vi "xijk_calc_other_parameters.vi"(7 "Settings":T1={"search parameters"={"Paths"={"Path: Excitation filters"=path "", "Path: Dicroic filters"=path "", "Path: Emission filters"=path "", "Path reget"=path ""}, "table excitation"=[], "table dicroics"=[], "table emission"=[], "Integers"={"Select result number"=1}, "boolean selector array"=[], "table for calculation automagic"=[]}, "output cluster"={"Booleans"={"Unknown detector"=FALSE, "Dual band filters"=FALSE, "Dual emission by cubes"=FALSE, "FRET"=FALSE}, "Integers"={"Light source"=0, "Number of fluorophores"=0, "Wavelength of laser (nm) 1"=0, "Broadness of laser (nm) 1"=0.0, "Wavelength of laser (nm) 2"=0, "Broadness of laser (nm) 2"=0.0, "Template"=1}, "Doubles"={"Molar extinction 1"=1.0, "Molar extinction 2"=1.0, "Quantum efficiency 1"=1.0, "Quantum efficiency 2"=1.0}}, "output cluster 2"={"Excitation filter 1"=path "", "Dichroic filter 1"=path "", "Emission filter 1"=path "", "Excitation filter 2"=path "", "Dichroic filter 2"=path "", "Emission filter 2"=path "", "Extra em filter 1"=path "", "Extra em filter 2"=path "", "Light source file"=path "", "Fluorophore absorption 1"=path "", "Fluorophore emission 1"=path "", "Fluorophore absorption 2"=path "", "Fluorophore emission 2"=path "", "Detector"=path ""}, "cluster de sortie"={"Excitation filter_x"=[], "Excitation filter_y"=[], "Dichroic filter_x"=[], "Dichroic filter_y"=[], "Emission filter_x"=[], "Emission filter_y"=[], "Excitation filter_x 2"=[], "Excitation filter_y 2"=[], "Dichroic filter_x 2"=[], "Dichroic filter_y 2"=[], "Emission filter_x 2"=[], "Emission filter_y 2"=[], "Extra em filter_x 1"=[], "Extra em filter_y 1"=[], "Extra em filter_x 1"=[], "Extra em filter_y 2"=[], "Light source_x"=[], "Light source_y"=[], "Detector_x"=[], "Detector_y"=[], "Fluorophore absorption_x"=[], "Fluorophore absorption_y"=[], "Fluorophore emission_x"=[], "Fluorophore emission_y"=[], "Fluorophore absorption_x 2"=[], "Fluorophore absorption_y 2"=[], "Fluorophore emission_x 2"=[], "Fluorophore emission_y 2"=[], "laser_x"=[], "laser_y"=[], "laser_x 2"=[], "laser_y 2"=[], "quantum efficiency factor 1"=0.0, "quantum efficiency factor 2"=0.0, "lamp scaling factor"=0.0}, "Xijk output cluster"={"Xijk 111"=0.0, "Xijk 112"=0.0, "Xijk 121"=0.0, "Xijk 122"=0.0, "Xijk 211"=0.0, "Xijk 212"=0.0, "Xijk 221"=0.0, "Xijk 222"=0.0, "Eijk 111"=0.0, "Eijk 112"=0.0, "Eijk 121"=0.0, "Eijk 122"=0.0, "Eijk 211"=0.0, "Eijk 212"=0.0, "Eijk 221"=0.0, "Eijk 222"=0.0}, "GUI configuration"={"axes in"={"min x-axis excitation"=300, "max x-axis excitation"=800, "min x-axis emission"=300, "max x-axis emission"=800, "precision of results"=2}, "plot colors in"={"Lanscape Portrait"=FALSE, "Plot logarithmic"=FALSE, "Ex/Em filters double"=FALSE, "Line colors"=[16734569, 56375, 16711916, 5896447, 16448250, 56375]}}, "references"={"Excitation filter 1 ref"=refnum, "Dichroic filter 1 ref"=refnum, "Emission filter 1 ref"=refnum, "Excitation filter 2 ref"=refnum, "Dichroic filter 2 ref"=refnum, "Emission filter 2 ref"=refnum, "Extra em filter 1 ref"=refnum, "Extra em filter 2 ref"=refnum, "Light source file ref"=refnum, "Fluorophore absorption 1 ref"=refnum, "Fluorophore emission 1 ref"=refnum, "Fluorophore absorption 2 ref"=refnum, "Fluorophore emission 2 ref"=refnum, "Detector ref"=refnum}} {"GUI configuration"."axes in"."precision of results" max=8 step=1}, 8 "Effective spectral emission 2":sgl[](array[numeric]), 9 "Effective spectral excitation 2":sgl[](array[numeric]), 10 "Effective spectral emission 1":sgl[](array[numeric]), 11 "Effective spectral excitation 1":sgl[](array[numeric])) -> (3 "array out":dbl[](array[numeric]))   [LabVIEW 2009]
uses:
  Type Def/settings.ctl
  Type Def/search_parameters.ctl
  Type Def/spectra_parameters.ctl
  Type Def/filepath.ctl
  Type Def/spectrum_table_control.ctl
  Type Def/xijk_cluster.ctl
  Type Def/configuration_cluster.ctl
  Type Def/axis_parameters.ctl
  Type Def/color_parameters.ctl
  Type Def/control_references_cluster.ctl
  <vilib>/Analysis/8numeric.llb/1D Numeric Integration.vi
  <vilib>/Analysis/NI_AALPro.lvlib
panel:
  out "% red emission in green channel":dbl
  out "spectral overlap efficiency":dbl
  out "% green emission in red channel":dbl
  out "excite %\nabsorption 2":dbl
  out "capture %\nemission 2":dbl
  out "excitation light bleed through 2":dbl caption="excitation light bleed through" format="%0.3e"
  out "excite %\nabsorption":dbl
  out "capture %\nemission":dbl
  out "excitation light bleed through":dbl format="%0.3e"
  # "Dichroic"
  # "Ex/Em filter"
  # "Fluorophore 1"
  # "Fluorophore 2"
  # "Laser /\nextra Em filter"
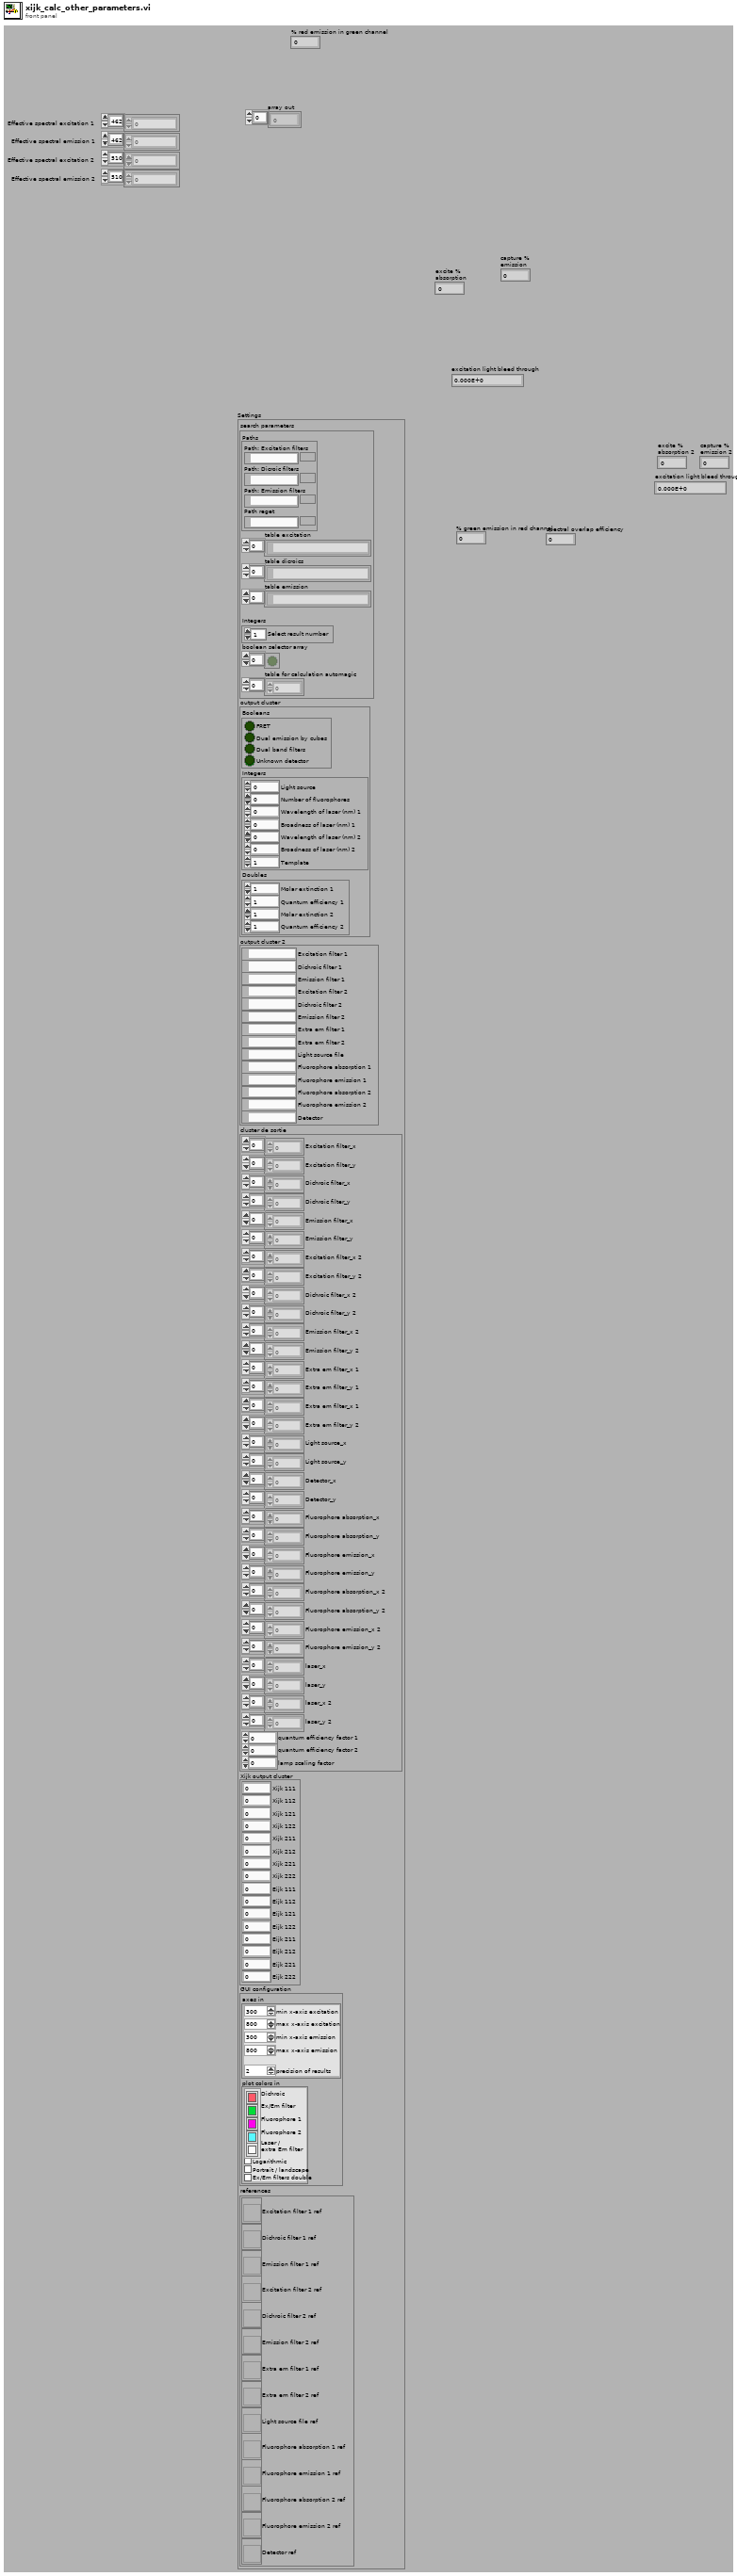
[diagram p1: front panel]
types:
  T1 = typedef "settings.ctl" = cluster{"search parameters":T2, "output cluster":T3, "output cluster 2":T4, "cluster de sortie":T5, "Xijk output cluster":T6, "GUI configuration":T7, "references":T10}
  T2 = typedef "search_parameters.ctl" = cluster{"Paths":cluster{"Path: Excitation filters":path, "Path: Dicroic filters":path, "Path: Emission filters":path, "Path reget":path}, "table excitation":path[], "table dicroics":path[], "table emission":path[], "Integers":cluster{"Select result number":u32}, "boolean selector array":bool[], "table for calculation automagic":i32[]}
  T3 = typedef "spectra_parameters.ctl" = cluster{"Booleans":cluster{"Unknown detector":bool, "Dual band filters":bool, "Dual emission by cubes":bool, "FRET":bool}, "Integers":cluster{"Light source":u16, "Number of fluorophores":u16, "Wavelength of laser (nm) 1":u16, "Broadness of laser (nm) 1":sgl, "Wavelength of laser (nm) 2":u16, "Broadness of laser (nm) 2":sgl, "Template":u16}, "Doubles":cluster{"Molar extinction 1":sgl, "Molar extinction 2":sgl, "Quantum efficiency 1":sgl, "Quantum efficiency 2":sgl}}
  T4 = typedef "filepath.ctl" = cluster{"Excitation filter 1":path, "Dichroic filter 1":path, "Emission filter 1":path, "Excitation filter 2":path, "Dichroic filter 2":path, "Emission filter 2":path, "Extra em filter 1":path, "Extra em filter 2":path, "Light source file":path, "Fluorophore absorption 1":path, "Fluorophore emission 1":path, "Fluorophore absorption 2":path, "Fluorophore emission 2":path, "Detector":path}
  T5 = typedef "spectrum_table_control.ctl" = cluster{"Excitation filter_x":i16[], "Excitation filter_y":sgl[], "Dichroic filter_x":i16[], "Dichroic filter_y":sgl[], "Emission filter_x":i16[], "Emission filter_y":sgl[], "Excitation filter_x 2":i16[], "Excitation filter_y 2":sgl[], "Dichroic filter_x 2":i16[], "Dichroic filter_y 2":sgl[], "Emission filter_x 2":i16[], "Emission filter_y 2":sgl[], "Extra em filter_x 1":i16[], "Extra em filter_y 1":sgl[], "Extra em filter_x 1":i16[], "Extra em filter_y 2":sgl[], "Light source_x":i16[], "Light source_y":sgl[], "Detector_x":i16[], "Detector_y":sgl[], "Fluorophore absorption_x":i16[], "Fluorophore absorption_y":sgl[], "Fluorophore emission_x":i16[], "Fluorophore emission_y":sgl[], "Fluorophore absorption_x 2":i16[], "Fluorophore absorption_y 2":sgl[], "Fluorophore emission_x 2":i16[], "Fluorophore emission_y 2":sgl[], "laser_x":i16[], "laser_y":sgl[], "laser_x 2":i16[], "laser_y 2":sgl[], "quantum efficiency factor 1":sgl, "quantum efficiency factor 2":sgl, "lamp scaling factor":sgl}
  T6 = typedef "xijk_cluster.ctl" = cluster{"Xijk 111":sgl, "Xijk 112":sgl, "Xijk 121":sgl, "Xijk 122":sgl, "Xijk 211":sgl, "Xijk 212":sgl, "Xijk 221":sgl, "Xijk 222":sgl, "Eijk 111":sgl, "Eijk 112":sgl, "Eijk 121":sgl, "Eijk 122":sgl, "Eijk 211":sgl, "Eijk 212":sgl, "Eijk 221":sgl, "Eijk 222":sgl}
  T7 = typedef "configuration_cluster.ctl" = cluster{"axes in":T8, "plot colors in":T9}
  T8 = typedef "axis_parameters.ctl" = cluster{"min x-axis excitation":u16, "max x-axis excitation":u16, "min x-axis emission":u16, "max x-axis emission":u16, "precision of results":u8}
  T9 = typedef "color_parameters.ctl" = cluster{"Lanscape Portrait":bool, "Plot logarithmic":bool, "Ex/Em filters double":bool, "Line colors":u32[]}
  T10 = typedef "control_references_cluster.ctl" = cluster{"Excitation filter 1 ref":refnum<vi>, "Dichroic filter 1 ref":refnum<vi>, "Emission filter 1 ref":refnum<vi>, "Excitation filter 2 ref":refnum<vi>, "Dichroic filter 2 ref":refnum<vi>, "Emission filter 2 ref":refnum<vi>, "Extra em filter 1 ref":refnum<vi>, "Extra em filter 2 ref":refnum<vi>, "Light source file ref":refnum<vi>, "Fluorophore absorption 1 ref":refnum<vi>, "Fluorophore emission 1 ref":refnum<vi>, "Fluorophore absorption 2 ref":refnum<vi>, "Fluorophore emission 2 ref":refnum<vi>, "Detector ref":refnum<vi>}
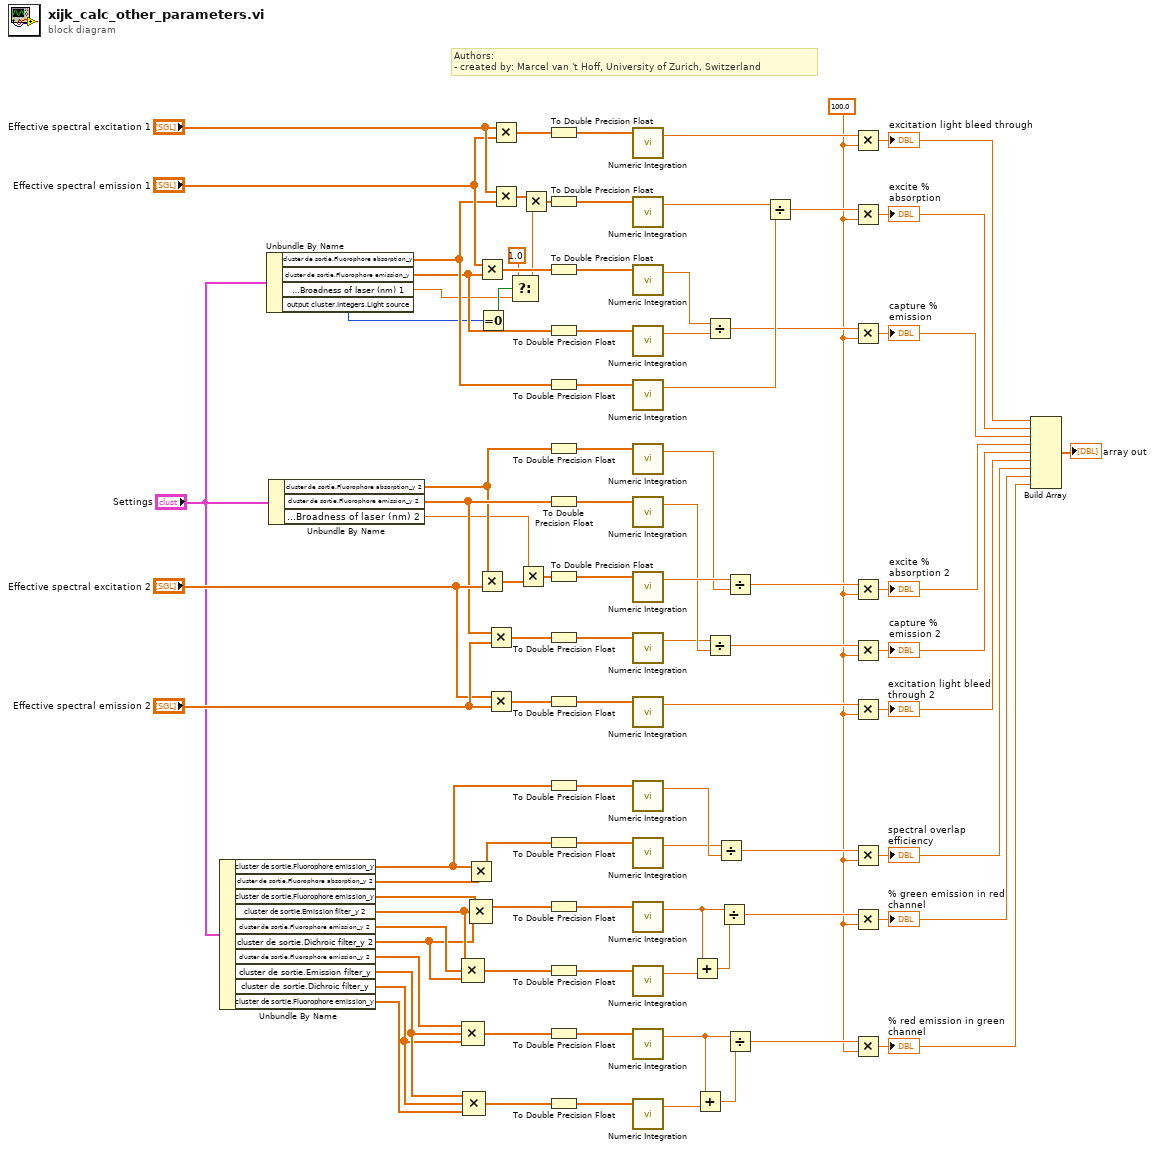
[diagram p0: block diagram]
diagram:
  w8 = 100.0 ("y")
  # "Authors: \n- created by: Marcel van 't Hoff, University of Zurich, Switzerland"
  n1 = Unbundle By Name("Settings") -> ("cluster de sortie.Fluorophore emission_y"=w32:sgl[], "cluster de sortie.Fluorophore absorption_y 2"=w65:sgl[], "cluster de sortie.Fluorophore emission_y"=w69:sgl[], "cluster de sortie.Emission filter_y 2"=w71:sgl[], "cluster de sortie.Fluorophore emission_y 2"=w70:sgl[], "cluster de sortie.Dichroic filter_y 2"=w55:sgl[], "cluster de sortie.Fluorophore emission_y 2"=w54:sgl[], "cluster de sortie.Emission filter_y"=w53:sgl[], "cluster de sortie.Dichroic filter_y"=w46:sgl[], "cluster de sortie.Fluorophore emission_y"=w47:sgl[])
  n2 = Unbundle By Name("Settings") -> ("cluster de sortie.Fluorophore absorption_y"=w20:sgl[], "cluster de sortie.Fluorophore emission_y"=w18:sgl[], "output cluster.Integers.Broadness of laser (nm) 1"=w2:sgl, "output cluster.Integers.Light source"=w1:u16)
  n3 = Unbundle By Name("Settings") -> ("cluster de sortie.Fluorophore absorption_y 2"=w22:sgl[], "cluster de sortie.Fluorophore emission_y 2"=w24:sgl[], "output cluster.Integers.Broadness of laser (nm) 2"=w3:sgl)
  n4 = Compound Arithmetic op=MULTIPLY(w71, w70, w55) -> (w38:sgl[])
  n5 = Compound Arithmetic op=MULTIPLY(w54, w53, w46) -> (w40:sgl[])
  n6 = Compound Arithmetic op=MULTIPLY(w53, w46, w47) -> (w52:sgl[])
  n7 = Multiply(x=w32, y=w65) -> (x*y=w34:sgl[])
  n8 = Compound Arithmetic op=MULTIPLY(w69, w71, w55) -> (w36:sgl[])
  n9 = Multiply(x="Effective spectral emission 1", y=w18) -> (x*y=w16:sgl[])
  n10 = Multiply(x=w22, y="Effective spectral excitation 2") -> (x*y=w81:sgl[])
  n11 = Equal To 0?(x=w1) -> (x = 0?=w7:bool)
  n12 = Multiply(x=w24, y="Effective spectral emission 2") -> (x*y=w28:sgl[])
  n13 = Multiply(x="Effective spectral excitation 2", y="Effective spectral emission 2") -> (x*y=w30:sgl[])
  n14 = Multiply(x="Effective spectral excitation 1", y="Effective spectral emission 1") -> (x*y=w12:sgl[])
  n15 = Multiply(x="Effective spectral excitation 1", y=w20) -> (x*y=w89:sgl[])
  n16 = Select(t=sgl 1.0, s=w7, f=w2) -> (s? t:f=w6:sgl)
  n17 = Multiply(x=w3, y=w81) -> (x*y=w26:sgl[])
  n18 = Multiply(x=w89, y=w6) -> (x*y=w14:sgl[])
  n19 = To Double Precision Float(number=w12) -> (double precision float=w11:dbl[])
  n20 = To Double Precision Float(number=w14) -> (double precision float=w13:dbl[])
  n21 = To Double Precision Float(number=w16) -> (double precision float=w15:dbl[])
  n22 = To Double Precision Float(number=w18) -> (double precision float=w17:dbl[])
  n23 = To Double Precision Float(number=w20) -> (double precision float=w19:dbl[])
  n24 = To Double Precision Float(number=w22) -> (double precision float=w21:dbl[])
  n25 = To Double Precision Float(number=w24) -> (double precision float=w23:dbl[])
  n26 = To Double Precision Float(number=w26) -> (double precision float=w25:dbl[])
  n27 = To Double Precision Float(number=w28) -> (double precision float=w27:dbl[])
  n28 = To Double Precision Float(number=w30) -> (double precision float=w29:dbl[])
  n29 = To Double Precision Float(number=w32) -> (double precision float=w31:dbl[])
  n30 = To Double Precision Float(number=w34) -> (double precision float=w33:dbl[])
  n31 = To Double Precision Float(number=w36) -> (double precision float=w35:dbl[])
  n32 = To Double Precision Float(number=w38) -> (double precision float=w37:dbl[])
  n33 = To Double Precision Float(number=w40) -> (double precision float=w39:dbl[])
  n34 = To Double Precision Float(number=w52) -> (double precision float=w41:dbl[])
  n35 = call-poly <vilib>:"Numeric Integration.vi"("Input Array"=w11) -> ("result"=w45:dbl)  [unwired: 2 in, 1 out]
  n36 = call-poly <vilib>:"Numeric Integration.vi"("Input Array"=w13) -> ("result"=w88:dbl)  [unwired: 2 in, 1 out]
  n37 = call-poly <vilib>:"Numeric Integration.vi"("Input Array"=w15) -> ("result"=w86:dbl)  [unwired: 2 in, 1 out]
  n38 = call-poly <vilib>:"Numeric Integration.vi"("Input Array"=w17) -> ("result"=w87:dbl)  [unwired: 2 in, 1 out]
  n39 = call-poly <vilib>:"Numeric Integration.vi"("Input Array"=w19) -> ("result"=w90:dbl)  [unwired: 2 in, 1 out]
  n40 = call-poly <vilib>:"Numeric Integration.vi"("Input Array"=w21) -> ("result"=w75:dbl)  [unwired: 2 in, 1 out]
  n41 = call-poly <vilib>:"Numeric Integration.vi"("Input Array"=w23) -> ("result"=w79:dbl)  [unwired: 2 in, 1 out]
  n42 = call-poly <vilib>:"Numeric Integration.vi"("Input Array"=w25) -> ("result"=w80:dbl)  [unwired: 2 in, 1 out]
  n43 = call-poly <vilib>:"Numeric Integration.vi"("Input Array"=w27) -> ("result"=w78:dbl)  [unwired: 2 in, 1 out]
  n44 = call-poly <vilib>:"Numeric Integration.vi"("Input Array"=w29) -> ("result"=w43:dbl)  [unwired: 2 in, 1 out]
  n45 = call-poly <vilib>:"Numeric Integration.vi"("Input Array"=w31) -> ("result"=w68:dbl)  [unwired: 2 in, 1 out]
  n46 = call-poly <vilib>:"Numeric Integration.vi"("Input Array"=w33) -> ("result"=w67:dbl)  [unwired: 2 in, 1 out]
  n47 = call-poly <vilib>:"Numeric Integration.vi"("Input Array"=w35) -> ("result"=w72:dbl)  [unwired: 2 in, 1 out]
  n48 = call-poly <vilib>:"Numeric Integration.vi"("Input Array"=w37) -> ("result"=w73:dbl)  [unwired: 2 in, 1 out]
  n49 = call-poly <vilib>:"Numeric Integration.vi"("Input Array"=w39) -> ("result"=w50:dbl)  [unwired: 2 in, 1 out]
  n50 = call-poly <vilib>:"Numeric Integration.vi"("Input Array"=w41) -> ("result"=w49:dbl)  [unwired: 2 in, 1 out]
  n51 = Add(x=w72, y=w73) -> (x+y=w74:dbl)
  n52 = Add(x=w50, y=w49) -> (x+y=w51:dbl)
  n53 = Divide(x=w86, y=w87) -> (x/y=w85:dbl)
  n54 = Divide(x=w78, y=w79) -> (x/y=w77:dbl)
  n55 = Divide(x=w67, y=w68) -> (x/y=w66:dbl)
  n56 = Divide(x=w72, y=w74) -> (x/y=w9:dbl)
  n57 = Divide(x=w80, y=w75) -> (x/y=w76:dbl)
  n58 = Divide(x=w50, y=w51) -> (x/y=w10:dbl)
  n59 = Divide(x=w88, y=w90) -> (x/y=w84:dbl)
  n60 = Multiply(x=w45, y=w8) -> (x*y=w44:dbl)
  "excitation light bleed through" <- w44
  n61 = Multiply(x=w84, y=w8) -> (x*y=w62:dbl)
  "excite %\nabsorption" <- w62
  n62 = Multiply(x=w85, y=w8) -> (x*y=w61:dbl)
  "capture %\nemission" <- w61
  n63 = Multiply(x=w76, y=w8) -> (x*y=w60:dbl)
  "excite %\nabsorption 2" <- w60
  n64 = Multiply(x=w77, y=w8) -> (x*y=w59:dbl)
  "capture %\nemission 2" <- w59
  n65 = Multiply(x=w43, y=w8) -> (x*y=w42:dbl)
  "excitation light bleed through 2" <- w42
  n66 = Multiply(x=w66, y=w8) -> (x*y=w58:dbl)
  "spectral overlap efficiency" <- w58
  n67 = Multiply(x=w9, y=w8) -> (x*y=w57:dbl)
  "% green emission in red channel" <- w57
  n68 = Multiply(x=w10, y=w8) -> (x*y=w48:dbl)
  "% red emission in green channel" <- w48
  n69 = Build Array(w44, w62, w61, w60, w59, w42, w58, w57, w48) -> (→"array out":dbl[])
